vi "piezoReadOpen.vi"   [LabVIEW 2017]
uses:
  globalDevices.vi
  <vilib>/DAQmx/create/channels.llb/DAQmx Create Channel (AI-Voltage-Basic).vi
  <vilib>/DAQmx/configure/timing.llb/DAQmx Timing (Sample Clock).vi
panel:
  # "Init VI for:\nReads the position of the piezo using the trigger of the Hamamatsu camera as clock."
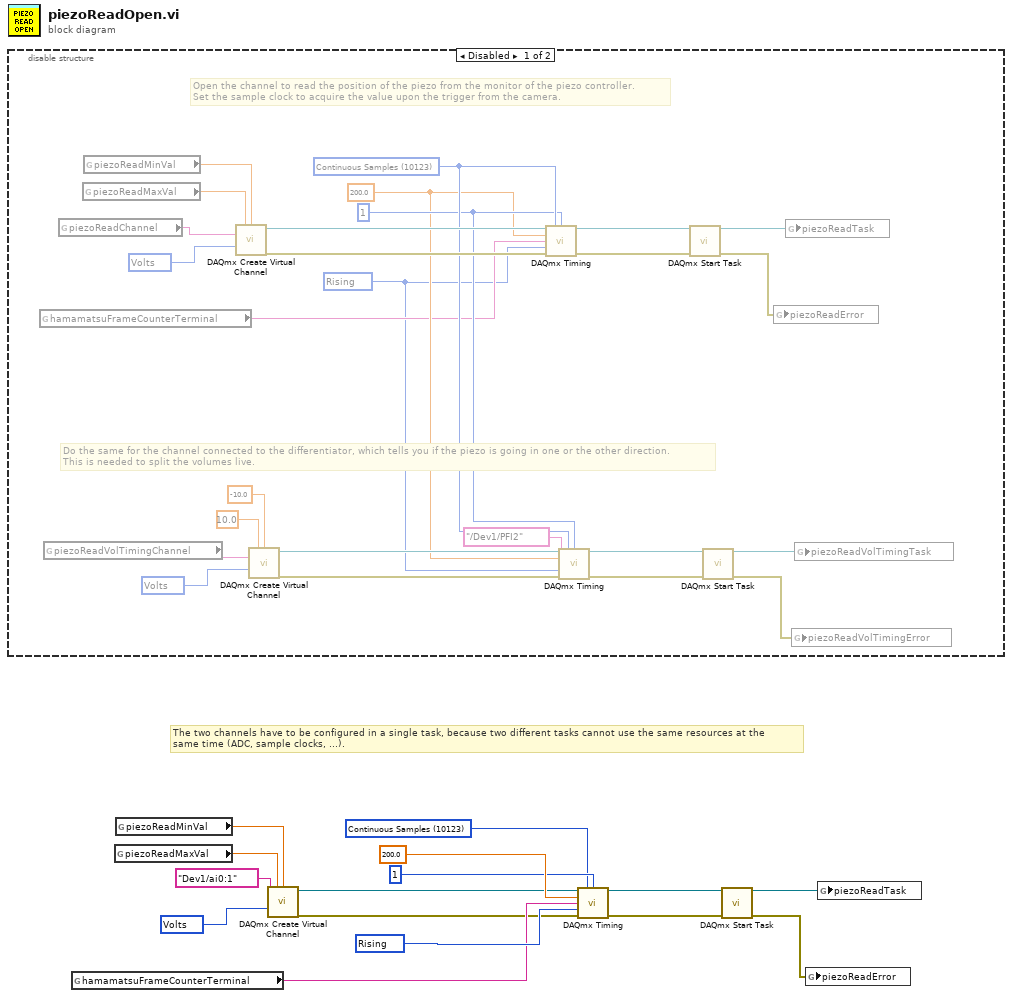
[diagram p0: block diagram]
diagram:
  w8 = 10348 items=["Volts"=10348, "From Custom Scale"=10065] ("units")
  w13 = 10280 items=["Rising"=10280, "Falling"=10171] ("active edge")
  w9 = 10123 items=["Finite Samples"=10178, "Continuous Samples"=10123, "Hardware Timed Single Point"=12522] ("sample mode")
  # "The two channels have to be configured in a single task, because two different tasks cannot use the same resources at the\nsame time (ADC, sample clocks, ...)."
  n1 = disable-structure shown="Disabled" {
    frame Disabled {
      w30 = 10348 items=["Volts"=10348, "From Custom Scale"=10065] ("units")
      w35 = 10348 items=["Volts"=10348, "From Custom Scale"=10065] ("units")
      w22 = 1 ("samples per channel")
      w19 = 10280 items=["Rising"=10280, "Falling"=10171] ("active edge")
      w21 = 200.0 ("rate")
      w23 = 10123 items=["Finite Samples"=10178, "Continuous Samples"=10123, "Hardware Timed Single Point"=12522] ("sample mode")
      # "Do the same for the channel connected to the differentiator, which tells you if the piezo is going in one or the other direction.\nThis is needed to split the volumes live."
      # "Open the channel to read the position of the piezo from the monitor of the piezo controller.\nSet the sample clock to acquire the value upon the trigger from the camera."
      n2 = global read "globalDevices.vi" "hamamatsuFrameCounterTerminal"() -> (w20:tag)
      n3 = global read "globalDevices.vi" "piezoReadVolTimingChannel"() -> (w33:tag)
      n4 = global read "globalDevices.vi" "piezoReadChannel"() -> (w34:tag)
      n5 = global read "globalDevices.vi" "piezoReadMaxVal"() -> (w18:dbl)
      n6 = global read "globalDevices.vi" "piezoReadMinVal"() -> (w17:dbl)
      n7 = call-poly <vilib>:"DAQmx Create Virtual Channel.vi"("maximum value"=w18, "minimum value"=w17, "physical channels"=w34, "units"=w35) -> ("task out"=w41:refnum<k21>, "error out"=w40:errorcluster)  [unwired: 10 in]
      n8 = call-poly <vilib>:"DAQmx Create Virtual Channel.vi"("maximum value"=10.0, "minimum value"=-10.0, "physical channels"=w33, "units"=w30) -> ("task out"=w24:refnum<k21>, "error out"=w25:errorcluster)  [unwired: 10 in]
      n9 = call-poly <vilib>:"DAQmx Timing.vi"("task/channels in"=w41, "sample mode"=w23, "samples per channel"=w22, "rate"=w21, "source"=w20, "active edge"=w19, "error in"=w40) -> ("task out"=w39:refnum<k21>, "error out"=w38:errorcluster)  [unwired: 7 in]
      n10 = call-poly <vilib>:"DAQmx Timing.vi"("task/channels in"=w24, "sample mode"=w23, "samples per channel"=w22, "rate"=w21, "source"=tag "/Dev1/PFI2", "active edge"=w19, "error in"=w25) -> ("task out"=w26:refnum<k21>, "error out"=w27:errorcluster)  [unwired: 7 in]
      n11 = call <vilib>:"DAQmx Start Task.vi"("task/channels in"=w39, "error in"=w38) -> ("task out"=w37:refnum<k21>, "error out"=w36:errorcluster)  [unwired: 12 in]
      n12 = call <vilib>:"DAQmx Start Task.vi"("task/channels in"=w26, "error in"=w27) -> ("task out"=w28:refnum<k21>, "error out"=w29:errorcluster)  [unwired: 12 in]
      n13 = global write "globalDevices.vi" "piezoReadError"(w36) -> ()
      n14 = global write "globalDevices.vi" "piezoReadTask"(w37) -> ()
      n15 = global write "globalDevices.vi" "piezoReadVolTimingError"(w29) -> ()
      n16 = global write "globalDevices.vi" "piezoReadVolTimingTask"(w28) -> ()
    }
    frame Enabled {
    }
  }
  n17 = global read "globalDevices.vi" "hamamatsuFrameCounterTerminal"() -> (w12:tag)
  n18 = global read "globalDevices.vi" "piezoReadMaxVal"() -> (w14:dbl)
  n19 = global read "globalDevices.vi" "piezoReadMinVal"() -> (w15:dbl)
  n20 = call-poly <vilib>:"DAQmx Create Virtual Channel.vi"("maximum value"=w14, "minimum value"=w15, "physical channels"=tag "Dev1/ai0:1", "units"=w8) -> ("task out"=w2:refnum<k21>, "error out"=w3:errorcluster)  [unwired: 10 in]
  n21 = call-poly <vilib>:"DAQmx Timing.vi"("task/channels in"=w2, "sample mode"=w9, "samples per channel"=1, "rate"=200.0, "source"=w12, "active edge"=w13, "error in"=w3) -> ("task out"=w4:refnum<k21>, "error out"=w5:errorcluster)  [unwired: 7 in]
  n22 = call <vilib>:"DAQmx Start Task.vi"("task/channels in"=w4, "error in"=w5) -> ("task out"=w6:refnum<k21>, "error out"=w7:errorcluster)  [unwired: 12 in]
  n23 = global write "globalDevices.vi" "piezoReadError"(w7) -> ()
  n24 = global write "globalDevices.vi" "piezoReadTask"(w6) -> ()
